vi "Load Subitems.vi"(7 "defer fp updates?(T)":bool=TRUE, 8 "error in (no error)":errorcluster, 9 "Tag":string, 11 "Application Data in":T1) -> (0 "error out":errorcluster, 1 "item children":string[](array[string]), 3 "Application Data out":T1)   [LabVIEW 2017, in "DSF Configuration Utility.lvlib"]
uses:
  DSF Configuration Utility.lvlib
  Source/Main VI/Application Data.ctl
  DSF Configuration API/1.0.0/Public/Controls/DSF Config Data RefNum.ctl
  Source/Main VI/Window State.ctl
  Source/Main VI/View Mode.ctl
  DSF Configuration API/1.0.0/Public/Read Item/Read Plugin.vi
  DSF Configuration API/1.0.0/Public/Read Item/Read Group.vi
  DSF Configuration API/1.0.0/Public/Read Item/Read Transfer.vi
  DSF Configuration API/1.0.0/DSF Configuration API.lvlib
panel:
  # "App\nData"
  # "App\nData"
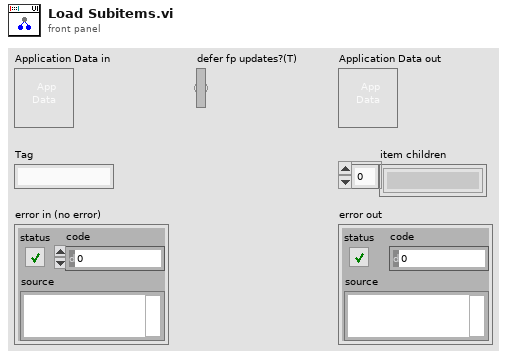
[diagram p1: front panel]
types:
  T1 = typedef "DSF Configuration Utility.lvlib/Application Data.ctl" = cluster{"DSF Refnum out":T2, "Tree Control":refnum<vi>, "Tab Control":refnum<vi>, "Top-Level VI":refnum<vi>, "value control refs":refnum<vi>[], "View State":T3}
  T2 = typedef "DSF Configuration API.lvlib/DSF Config Data RefNum.ctl" = refnum<k1>
  T3 = typedef "DSF Configuration Utility.lvlib/View Mode.ctl" = enum16{"Tree", "List"}
  T4 = typedef "DSF Configuration Utility.lvlib/Tree Item Type.ctl" = enum16{"Plugin", "Group", "Transfer", "Channel", "Setting"}
  T5 = typedef "DSF Configuration API.lvlib/DSF Plugin Info.ctl" = cluster{"type":string, "timing":T6, "group ids":string[], "settings id":string}
  T6 = typedef "DSF Configuration API.lvlib/DSF Timing Info.ctl" = cluster{"decimation":i32, "offset":i32}
  T7 = typedef "DSF Configuration Utility.lvlib/Tree Item.ctl" = cluster{"Left Cell String":string, "Child Text":string[], "Child Tag":string, "Glyph Index":i32}
  T8 = typedef "DSF Configuration API.lvlib/DSF Group Info.ctl" = cluster{"direction":i32, "timing":T6, "transfer ids":string[], "settings id":string}
  T9 = typedef "DSF Configuration API.lvlib/DSF Transfer Info.ctl" = cluster{"byte order":i32, "channel ids":string[], "settings id":string}
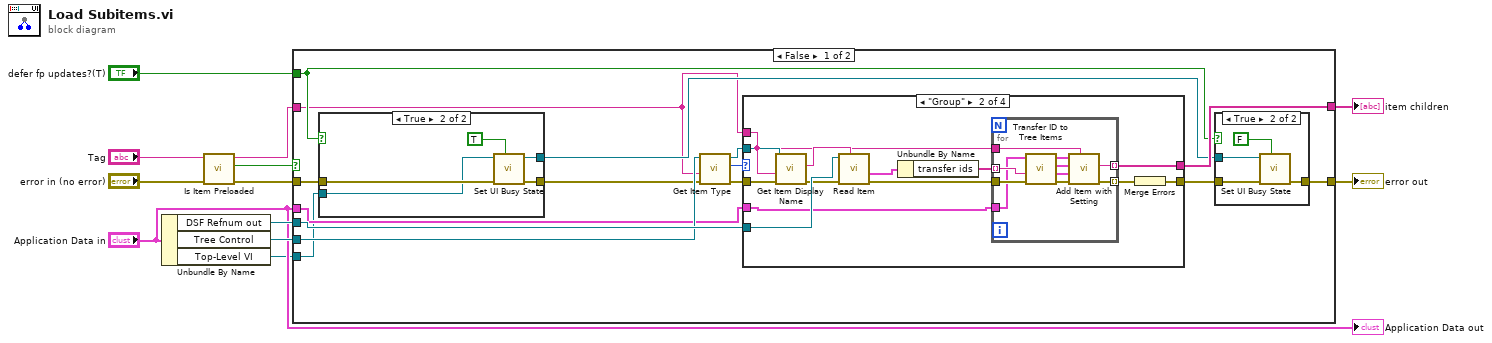
[diagram p0: block diagram]
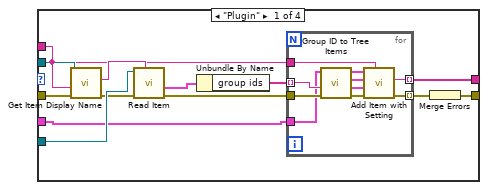
[diagram p4: hidden frame]
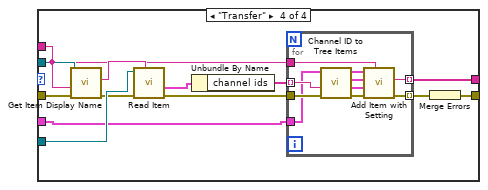
[diagram p6: hidden frame]
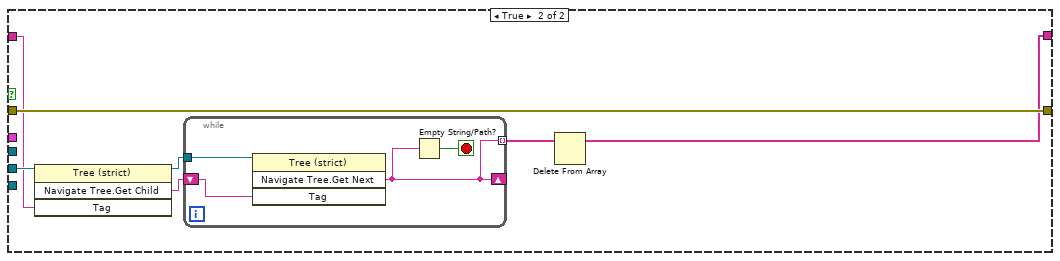
[diagram p7: hidden frame]
diagram:
  n1 = Unbundle By Name("Application Data in") -> ("DSF Refnum out"=w5:T2, "Tree Control"=w4:refnum<vi>, "Top-Level VI"=w2:refnum<vi>)
  n2 = call "Is Item Preloaded"("error in (no error)"="error in (no error)", "Tag in"="Tag") -> ("error out"=w9:errorcluster, "replaced"=w11:bool, "Tag out"=w12:string)  [unwired: 7 in]
  n3 = case shown="False" w11 {
    tunnel: w5 -> [w26 _]
    tunnel: w4 -> [w23 w114]
    tunnel: [w16 w115] -> w8
    tunnel: w9 -> [w22 w115]
    tunnel: w12 -> [w13 w113]
    tunnel: [w21 w110] -> w6
    tunnel: "Application Data in" -> [w19 _]
    tunnel: w2 -> [w18 _]
    tunnel: "defer fp updates?(T)" -> [w14 _]
    frame False {
      n4 = case shown="True" w14 {
        tunnel: w22 -> [w33 w38]
        tunnel: w18 -> [_ w37]
        tunnel: [w33 w36] -> w17
        tunnel: [_ w35] -> w15
        frame False {
        }
        frame True {
          n5 = call "Set UI Busy State.vi"("Defer Panel Updates"=TRUE, "error in (no error)"=w38, "VI in"=w37) -> ("error out"=w36:errorcluster, "VI out"=w35:refnum<vi>)  [unwired: 7 in]
        }
      }
      n6 = call "Get Item Type.vi"("error in (no error)"=w17, "Tag"=w13, "TreeControl in"=w23) -> ("error out"=w27:errorcluster, "Item Type"=w25:T4, "TreeControl out"=w20:refnum<vi>)  [unwired: 6 in]
      n7 = case shown="\"Group\"" w25 {
        tunnel: w20 -> [w51 w74 _ w98]
        tunnel: w27 -> [w50 w73 w85 w97]
        tunnel: w26 -> [w49 w72 _ w96]
        tunnel: [w43 w66 w85 w91] -> w24
        tunnel: w13 -> [w39 w62 _ w86]
        tunnel: [w41 w64 _ w88] -> w21
        tunnel: w19 -> [w40 w63 _ w87]
        frame "Plugin" {
          n8 = call "Get Item Display Name.vi"("error in (no error)"=w50, "Tag"=w39, "TreeControl in"=w51) -> ("error out"=w48:errorcluster, "display name"=w42:string)  [unwired: 6 in, 1 out]
          n9 = call-poly "Read Item.vi"("name"=w42, "error in (no error)"=w48, "refnum"=w49) -> ("error out"=w45:errorcluster, "value"=w47:T5)  [unwired: 5 in, 2 out]
          n10 = Unbundle By Name(w47) -> ("group ids"=w46:string[])
          n11 = for {
            tunnel: w46 -> [w61] mode=indexing
            tunnel: w45 -> [w60]
            tunnel: [w58] -> w44 mode=indexing
            tunnel: w39 -> [w53]
            tunnel: [w56] -> w41 mode=indexing
            tunnel: w40 -> [w55]
            n12 = call "Group ID to Tree Items.vi"("error in (no error)"=w60, "Group ID"=w61, "Application Data in"=w55) -> ("error out"=w59:errorcluster, "Settings"=w52:T7, "Item"=w57:T7, "Application Data out"=w54:T1)  [unwired: 5 in]
            n13 = call "Add Item with Setting.vi"("Tag"=w53, "error in (no error)"=w59, "Setting"=w52, "Item"=w57, "Application Data in"=w54) -> ("error out"=w58:errorcluster, "new item tag"=w56:string)  [unwired: 4 in, 1 out]
          }
          n14 = Merge Errors(w44) -> (w43:errorcluster)
        }
        frame "Group" {
          n15 = call "Get Item Display Name.vi"("error in (no error)"=w73, "Tag"=w62, "TreeControl in"=w74) -> ("error out"=w71:errorcluster, "display name"=w67:string)  [unwired: 6 in, 1 out]
          n16 = call-poly "Read Item.vi"("name"=w67, "error in (no error)"=w71, "refnum"=w72) -> ("error out"=w68:errorcluster, "value"=w70:T8)  [unwired: 5 in, 2 out]
          n17 = Unbundle By Name(w70) -> ("transfer ids"=w69:string[])
          n18 = for {
            tunnel: w69 -> [w84] mode=indexing
            tunnel: w68 -> [w83]
            tunnel: [w81] -> w65 mode=indexing
            tunnel: w62 -> [w77]
            tunnel: [w80] -> w64 mode=indexing
            tunnel: w63 -> [w78]
            n19 = call "Transfer ID to Tree Items.vi"("error in (no error)"=w83, "Transfer ID"=w84, "Application Data in"=w78) -> ("error out"=w82:errorcluster, "Settings"=w75:T7, "Item"=w76:T7, "Application Data out"=w79:T1)  [unwired: 5 in]
            n20 = call "Add Item with Setting.vi"("Tag"=w77, "error in (no error)"=w82, "Setting"=w75, "Item"=w76, "Application Data in"=w79) -> ("error out"=w81:errorcluster, "new item tag"=w80:string)  [unwired: 4 in, 1 out]
          }
          n21 = Merge Errors(w65) -> (w66:errorcluster)
        }
        frame "Channel", "Setting" {
        }
        frame "Transfer" {
          n22 = call "Get Item Display Name.vi"("error in (no error)"=w97, "Tag"=w86, "TreeControl in"=w98) -> ("error out"=w95:errorcluster, "display name"=w92:string)  [unwired: 6 in, 1 out]
          n23 = call-poly "Read Item.vi"("name"=w92, "error in (no error)"=w95, "refnum"=w96) -> ("error out"=w93:errorcluster, "value"=w94:T9)  [unwired: 5 in, 2 out]
          n24 = Unbundle By Name(w94) -> ("channel ids"=w89:string[])
          n25 = for {
            tunnel: w89 -> [w108] mode=indexing
            tunnel: w93 -> [w107]
            tunnel: [w105] -> w90 mode=indexing
            tunnel: w86 -> [w101]
            tunnel: [w104] -> w88 mode=indexing
            tunnel: w87 -> [w103]
            n26 = call "Channel ID to Tree Items.vi"("error in (no error)"=w107, "Channel ID"=w108, "Application Data in"=w103) -> ("error out"=w106:errorcluster, "Settings"=w100:T7, "Item"=w99:T7, "Application Data out"=w102:T1)  [unwired: 5 in]
            n27 = call "Add Item with Setting.vi"("Tag"=w101, "error in (no error)"=w106, "Setting"=w100, "Item"=w99, "Application Data in"=w102) -> ("error out"=w105:errorcluster, "new item tag"=w104:string)  [unwired: 4 in, 1 out]
          }
          n28 = Merge Errors(w90) -> (w91:errorcluster)
        }
      }
      n29 = case shown="True" w14 {
        tunnel: w24 -> [w28 w32]
        tunnel: [w28 w31] -> w16
        tunnel: w15 -> [_ w30]
        frame False {
        }
        frame True {
          n30 = call "Set UI Busy State.vi"("Defer Panel Updates"=FALSE, "error in (no error)"=w32, "VI in"=w30) -> ("error out"=w31:errorcluster)  [unwired: 7 in, 1 out]
        }
      }
    }
    frame True {
      n31 = invoke class="Tree (strict)" method="Navigate Tree.Get Child"(reference=w114, "Tag"=w113) -> (reference out=w112:refnum<vi>, "Navigate Tree:Get Child"=w109:string)  [unwired: 2 in, 2 out]
      n32 = while {
        tunnel: w112 -> [w119]
        tunnel: [w116] -> w111 mode=indexing
        shift-right: [w116] -> _
        shift-left: w109 -> [w117]
        stop <- w118 stop-if-true
        n33 = invoke class="Tree (strict)" method="Navigate Tree.Get Next"(reference=w119, "Tag"=w117) -> ("Navigate Tree:Get Next Item"=w116:string)  [unwired: 2 in, 3 out]
        n34 = Empty String/Path?(string/path=w116) -> (empty?=w118:bool)
      }
      n35 = Delete From Array(array=w111) -> (array with subset deleted=w110:string[])  [unwired: 2 in, 1 out]
    }
  }
  "error out" <- w8
  "item children" <- w6
  "Application Data out" <- "Application Data in"
